vi "GetBarValue.vi"(8 "error in (no error)":errorcluster, 11 "MGI_Progress Bar in":refnum<class "Progress Bar.lvclass">) -> (0 "error out":errorcluster, 2 "Progress Bar Value (0-100)":dbl, 3 "MGI_Progress Bar out":refnum<class "Progress Bar.lvclass">)   [LabVIEW 2020, in "Progress Bar.lvclass"]
doc: "Returns Current Iterations/ Total iterations. Override this VI if you want to use a different calculation\n\nCopyright: MGI\nAuthored by: Derek Trepanier"
uses:
  <userlib>/_MGI/User Interface/Progress Bar/Progress Bar.lvclass
  <userlib>/_MGI/User Interface/Progress Bar/Progress Bar.lvclass/Progress Bar.ctl
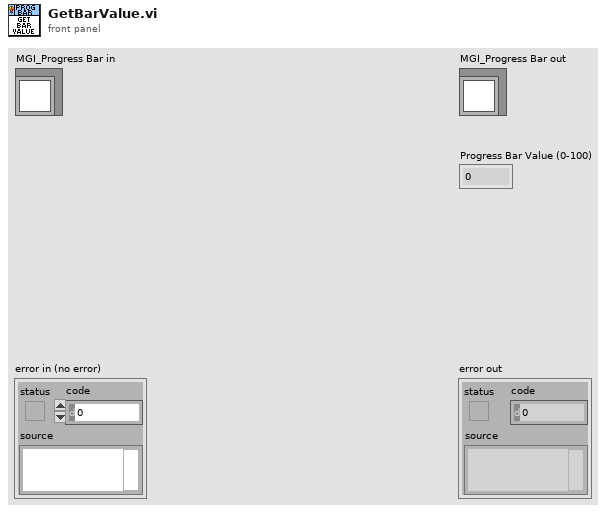
[diagram p1: front panel]
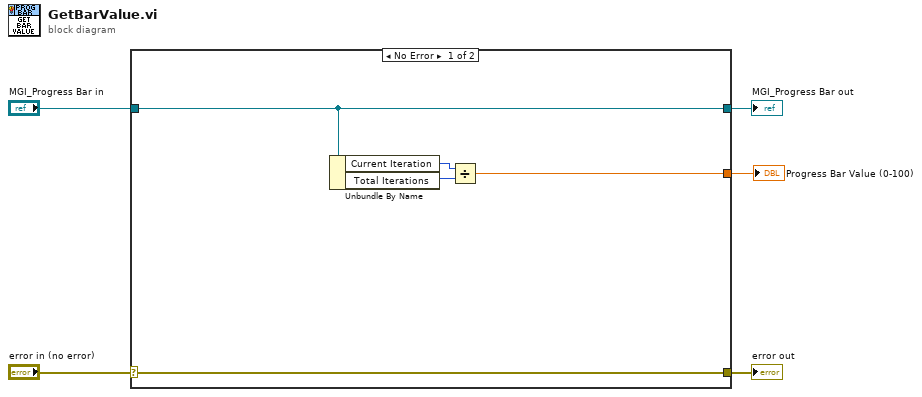
[diagram p0: block diagram]
diagram:
  n1 = case shown="No Error" "error in (no error)" {
    selector: "error in (no error)" -> [w10 w12]
    tunnel: [w10 w12] -> w4
    tunnel: [w9 w11] -> w2
    tunnel: "MGI_Progress Bar in" -> [w9 w11]
    tunnel: [w6 _] -> w1
    frame No Error {
      n2 = Unbundle By Name(w9) -> ("Current Iteration"=w8:i32, "Total Iterations"=w7:i32)
      n3 = Divide(x=w8, y=w7) -> (x/y=w6:dbl)
    }
    frame Error {
    }
  }
  "error out" <- w4
  "MGI_Progress Bar out" <- w2
  "Progress Bar Value (0-100)" <- w1
